vi "SquareWave.vi"(7 "Sample Rate":dbl, 8 "Sawtooth Wave DC Offset":dbl=4.0 format="%0.2f", 9 "Sawtooth Wave Amplitude":dbl=3.0 format="%0.2f", 10 "Sawtooth Wave Duration":dbl=20.0 format="%.2f", 11 "Sawtooth Wave Oscillations":dbl=10.0 format="%.2f") -> (1 "Frequency":dbl=0.5 format="%.2f", 2 "signal":dbl[](array[numeric]))   [LabVIEW 2016]
uses:
  <vilib>/Analysis/NI_AALPro.lvlib
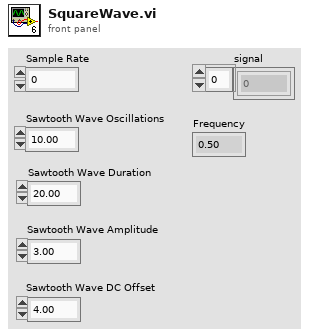
[diagram p1: front panel]
types:
  T1 = enum16{"sine", "cosine", "triangle", "square", "sawtooth", "increasing ramp", "decreasing ramp"}
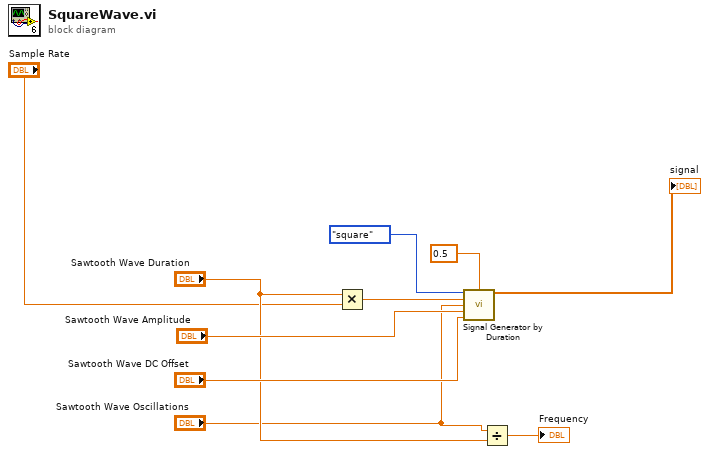
[diagram p0: block diagram]
diagram:
  n1 = Multiply(x="Sawtooth Wave Duration", y="Sample Rate") -> (x*y=w2:dbl)
  n2 = call <vilib>:"Signal Generator by Duration.vi"("signal type"=T1."square" ("waveform type"), "duration"=0.5, "# of samples"=w2, "frequency"="Sawtooth Wave Oscillations", "amplitude"="Sawtooth Wave Amplitude", "dc offset"="Sawtooth Wave DC Offset") -> ("signal"=→"signal":dbl[])  [unwired: 6 in, 3 out]
  n3 = Divide(x="Sawtooth Wave Oscillations", y="Sawtooth Wave Duration") -> (x/y=→"Frequency":dbl)
